vi "Calculate Plating Time.vi"(6 "Num Steps":i32, 9 "ItemNames":string[][](array[string]), 10 "Reverse Current Multiplier":dbl) -> (2 "Right Anode Time":dbl, 3 "Left Anode Time":dbl)   [LabVIEW 2019]
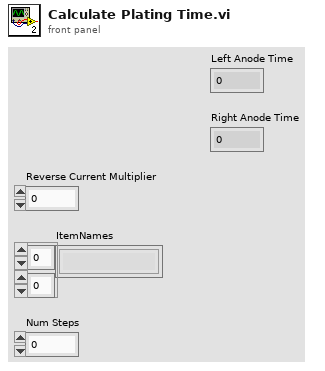
[diagram p1: front panel]
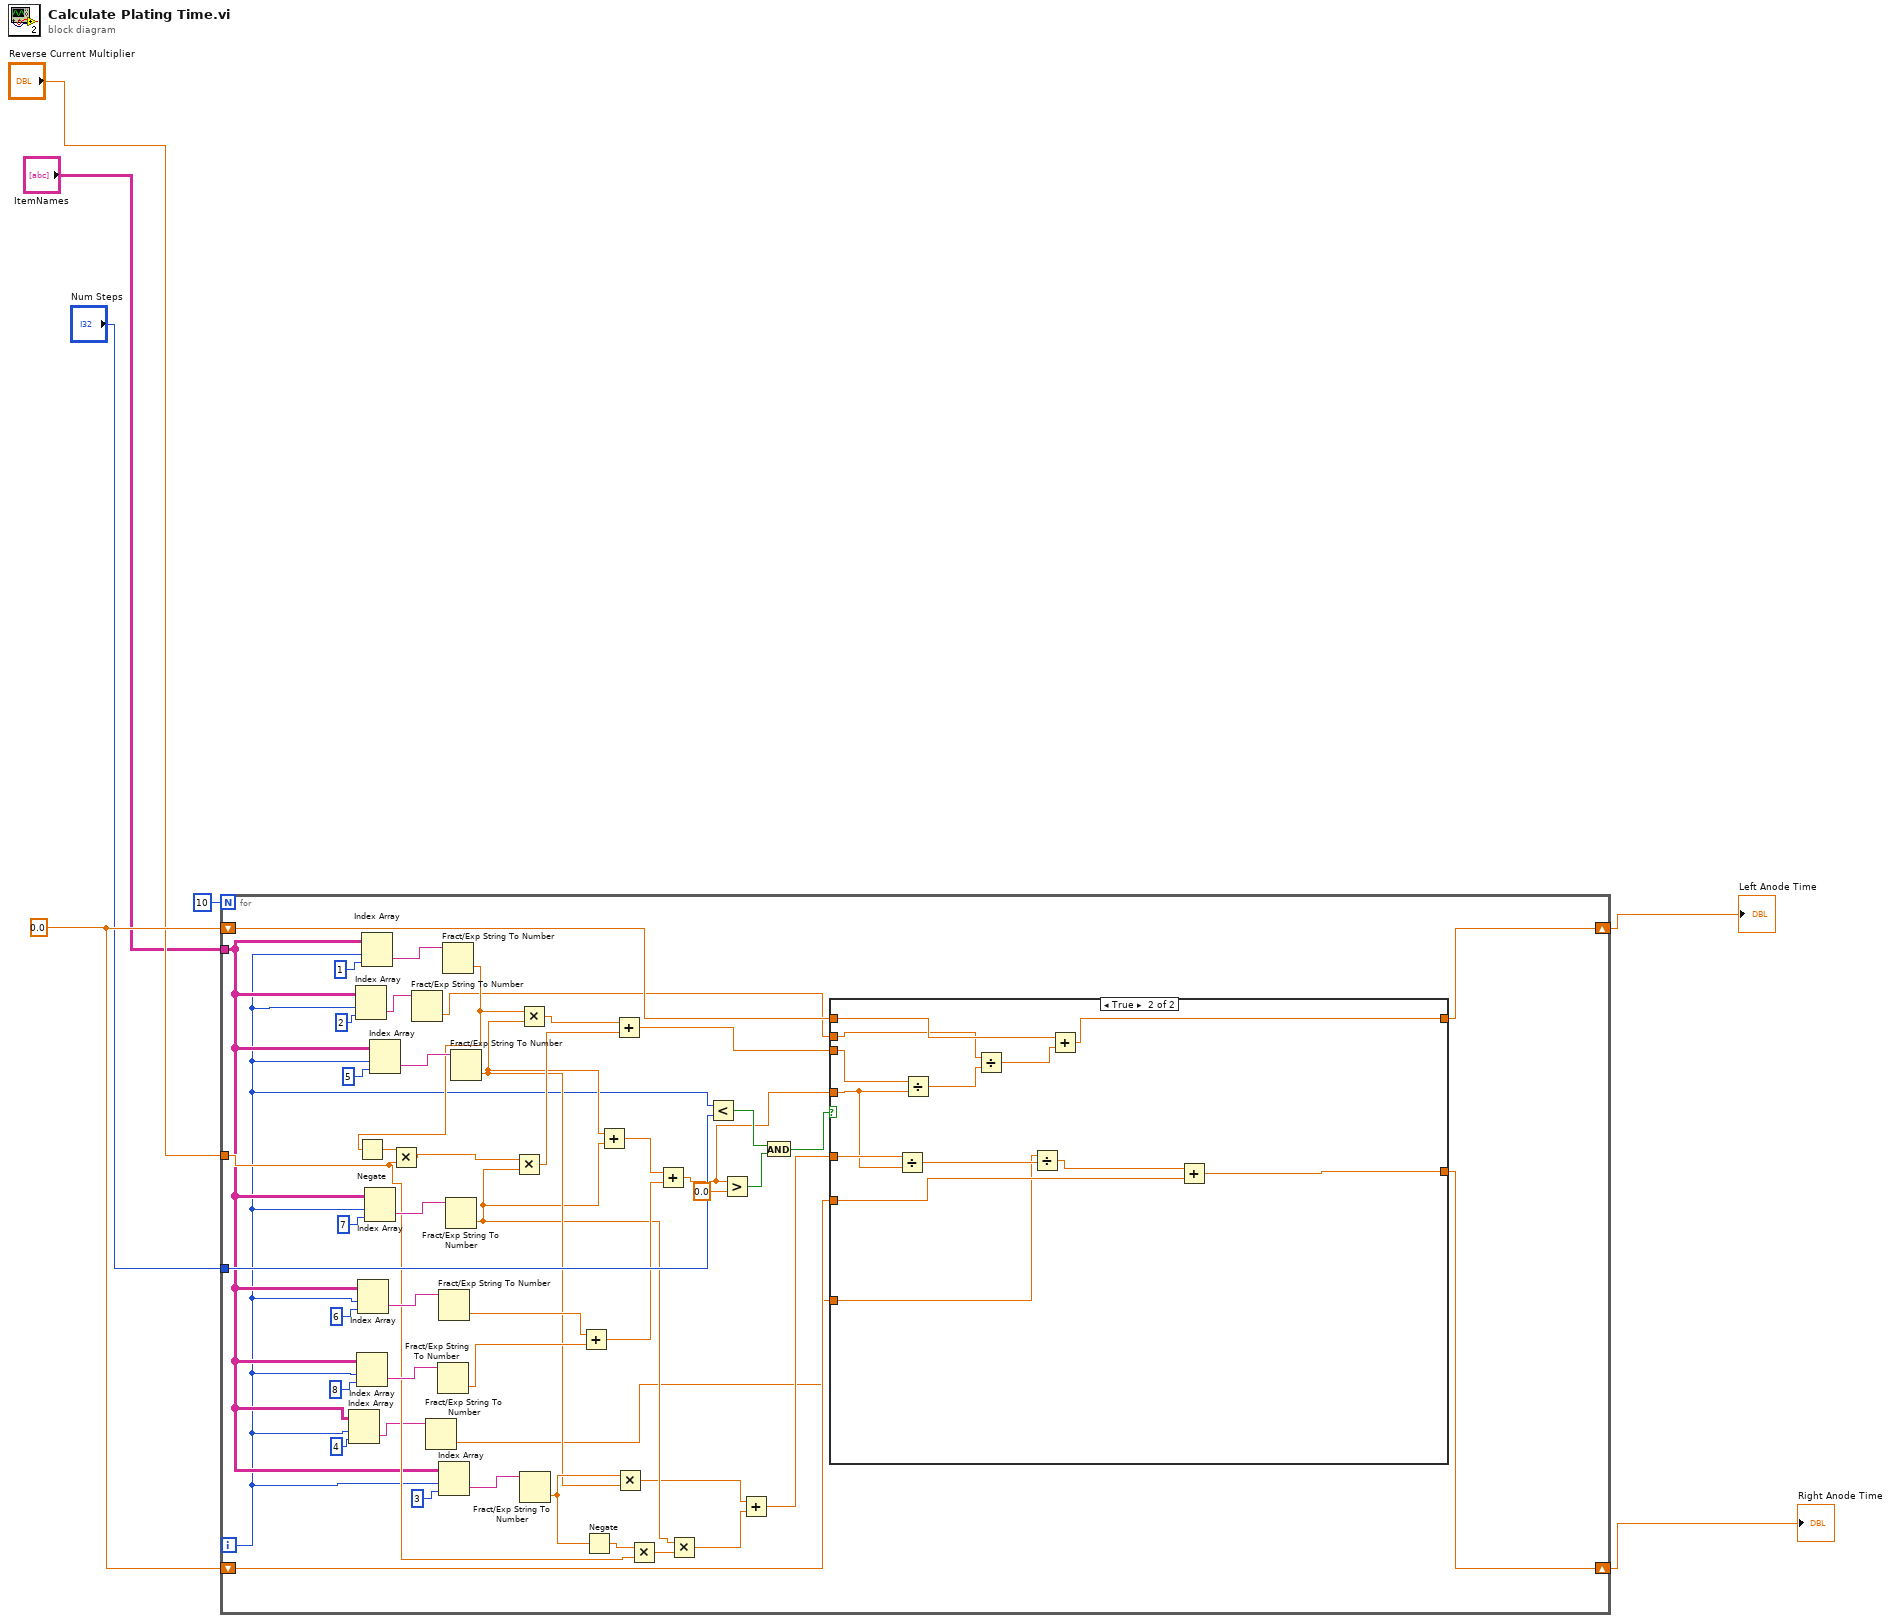
[diagram p0: block diagram]
diagram:
  w7 = 0.0 ("Numeric 3")
  n1 = for {
    N: 10 -> [_]
    tunnel: "ItemNames" -> [w10]
    tunnel: "Reverse Current Multiplier" -> [w23]
    tunnel: "Num Steps" -> [w45]
    shift-right: [w30] -> w1
    shift-left: w7 -> [w31]
    shift-right: [w16] -> w2
    shift-left: w7 -> [w17]
    i -> [w9]
    n2 = Index Array(array=w10, index (row)=w9, index (col)=4 ("disabled index (col)")) -> (element=w11:string)
    n3 = Index Array(array=w10, index (row)=w9, index (col)=2 ("disabled index (col)")) -> (element=w15:string)
    n4 = Index Array(array=w10, index (row)=w9, index (col)=8 ("disabled index (col)")) -> (element=w40:string)
    n5 = Index Array(array=w10, index (row)=w9, index (col)=6 ("disabled index (col)")) -> (element=w42:string)
    n6 = Index Array(array=w10, index (row)=w9, index (col)=1 ("disabled index (col)")) -> (element=w55:string)
    n7 = Index Array(array=w10, index (row)=w9, index (col)=7 ("disabled index (col)")) -> (element=w51:string)
    n8 = Index Array(array=w10, index (row)=w9, index (col)=5 ("disabled index (col)")) -> (element=w53:string)
    n9 = Fract/Exp String To Number(string=w15) -> (number=w13:dbl)  [unwired: 3 in, 1 out]
    n10 = Fract/Exp String To Number(string=w11) -> (number=w8:dbl)  [unwired: 3 in, 1 out]
    n11 = Fract/Exp String To Number(string=w40) -> (number=w38:dbl)  [unwired: 3 in, 1 out]
    n12 = Fract/Exp String To Number(string=w42) -> (number=w39:dbl)  [unwired: 3 in, 1 out]
    n13 = Index Array(array=w10, index (row)=w9, index (col)=3 ("disabled index (col)")) -> (element=w27:string)
    n14 = Fract/Exp String To Number(string=w55) -> (number=w50:dbl)  [unwired: 3 in, 1 out]
    n15 = Negate(x=w50) -> (-x=w49:dbl)
    n16 = Multiply(x=w49, y=w23) -> (x*y=w48:dbl)
    n17 = Fract/Exp String To Number(string=w51) -> (number=w21:dbl)  [unwired: 3 in, 1 out]
    n18 = Fract/Exp String To Number(string=w53) -> (number=w25:dbl)  [unwired: 3 in, 1 out]
    n19 = Multiply(x=w48, y=w21) -> (x*y=w46:dbl)
    n20 = Multiply(x=w50, y=w25) -> (x*y=w47:dbl)
    n21 = Fract/Exp String To Number(string=w27) -> (number=w26:dbl)  [unwired: 3 in, 1 out]
    n22 = Add(x=w39, y=w38) -> (x+y=w36:dbl)
    n23 = Negate(x=w26) -> (-x=w24:dbl)
    n24 = Add(x=w25, y=w21) -> (x+y=w37:dbl)
    n25 = Add(x=w47, y=w46) -> (x+y=w44:dbl)
    n26 = Multiply(x=w26, y=w25) -> (x*y=w20:dbl)
    n27 = Multiply(x=w24, y=w23) -> (x*y=w22:dbl)
    n28 = Add(x=w37, y=w36) -> (x+y=w29:dbl)
    n29 = Multiply(x=w21, y=w22) -> (x*y=w19:dbl)
    n30 = Less?(x=w9, y=w45) -> (x < y?=w34:bool)
    n31 = Greater?(x=w29, y=0.0) -> (0:w33:bool)
    n32 = Add(x=w20, y=w19) -> (x+y=w18:dbl)
    n33 = And(x=w34, y=w33) -> (x .and. y?=w32:bool)
    n34 = case shown="True" w32 {
      tunnel: w44 -> [_ w70]
      tunnel: w31 -> [w58 w71]
      tunnel: [w58 w69] -> w30
      tunnel: w29 -> [_ w67]
      tunnel: w18 -> [_ w68]
      tunnel: w17 -> [w57 w66]
      tunnel: [w57 w65] -> w16
      tunnel: w13 -> [_ w63]
      tunnel: w8 -> [_ w60]
      frame False {
      }
      frame True {
        n35 = Divide(x=w68, y=w67) -> (x/y=w61:dbl)
        n36 = Divide(x=w70, y=w67) -> (x/y=w64:dbl)
        n37 = Divide(x=w63, y=w64) -> (x/y=w62:dbl)
        n38 = Divide(x=w60, y=w61) -> (x/y=w59:dbl)
        n39 = Add(x=w71, y=w62) -> (x+y=w69:dbl)
        n40 = Add(x=w59, y=w66) -> (x+y=w65:dbl)
      }
    }
  }
  "Right Anode Time" <- w2
  "Left Anode Time" <- w1
